vi "Write.vi"(8 "error in (no error)":errorcluster, 9 "Data":u8[](array[numeric]) format="%.0x", 10 "Address":u8 format="%.0x", 11 "I2C Bus In":refnum<class "Mock I2C Bus.lvclass">) -> (0 "error out":errorcluster, 3 "I2C Bus Out":refnum<class "Mock I2C Bus.lvclass">)   [LabVIEW 2020, in "Mock I2C Bus.lvclass"]
uses:
  Mock I2C Bus.lvclass
  C:/Program Files (x86)/National Instruments/LabVIEW 2020/vi.lib/Astemes/LMock/Mock.lvclass
  <vilib>/Astemes/LMock/Mock.lvclass
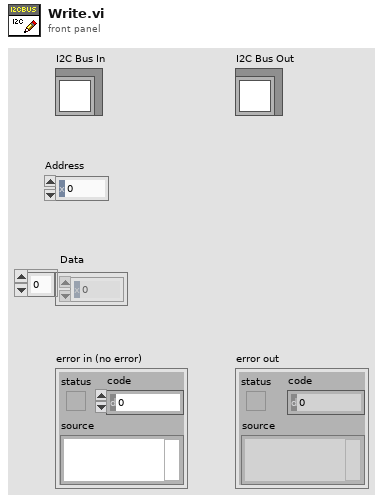
[diagram p1: front panel]
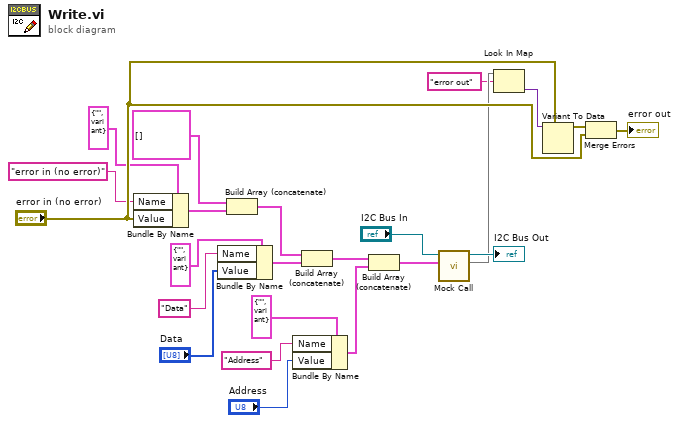
[diagram p0: block diagram]
diagram:
  n1 = Bundle By Name(cluster=cluster{"Name":string, "Value":variant} {"Name"="", "Value"=variant} ("element"), "Name"="error in (no error)", "Value"="error in (no error)") -> (w5:cluster{"Name":string, "Value":variant})
  n2 = Bundle By Name(cluster=cluster{"Name":string, "Value":variant} {"Name"="", "Value"=variant} ("element"), "Name"="Data", "Value"="Data") -> (w3:cluster{"Name":string, "Value":variant})
  n3 = Build Array (concatenate)(cluster{"Name":string, "Value":variant}[] [] ("Control Values"), w5) -> (w14:cluster{"Name":string, "Value":variant}[])
  n4 = Bundle By Name(cluster=cluster{"Name":string, "Value":variant} {"Name"="", "Value"=variant} ("element"), "Name"="Address", "Value"="Address") -> (w1:cluster{"Name":string, "Value":variant})
  n5 = Build Array (concatenate)(w14, w3) -> (w17:cluster{"Name":string, "Value":variant}[])
  n6 = Build Array (concatenate)(w17, w1) -> (w20:cluster{"Name":string, "Value":variant}[])
  n7 = call <vilib>:"Mock Call.vi"("Control Values"=w20, "Mock In"="I2C Bus In") -> ("Return Values"=w12:map{string, variant}, "Mock Out"=→"I2C Bus Out":refnum<class "Mock I2C Bus.lvclass">)  [unwired: 8 in]
  n8 = Look In Map(map=w12, key="error out") -> (value=w10:variant)  [unwired: 1 in, 1 out]
  n9 = Variant To Data(type="error in (no error)", Variant=w10) -> (data=w9:errorcluster)  [unwired: 1 in, 1 out]
  n10 = Merge Errors(w9, "error in (no error)") -> (→"error out":errorcluster)
